vi "WriteBusDataToFile.vi"(8 "ErrorArray In":errorcluster[](array[cluster]), 10 "Bus.lvclass In":refnum<class "Bus.lvclass">, 11 "TestFileRef In":T1) -> (0 "ErrorArray Out":errorcluster[](array[cluster]), 2 "Bus.lvclass Out":refnum<class "Bus.lvclass">, 3 "TestFileRef Out":T1)   [LabVIEW 2017, in "Bus_class.lvlib" / "Bus.lvclass"]
uses:
  Bus.lvclass
  <vilib>/Utility/config.llb/Config Data RefNum.ctl
  TypeDefs/clBusData.ctl
  FrontPanel/TypeDefs/clEventConfig.ctl
  Modules/PmuImpairPlugins/PmuImpairPluginBase_class/TypeDefs/clImpairConfig.ctl
  Modules/EventPlugins/EventPluginBaseClass/TypeDefs/clEvtReportArray.ctl
  Modules/EventPlugins/EventPluginBaseClass/TypeDefs/clEvtReport.ctl
  Modules/EventPlugins/EventPluginBaseClass/TypeDefs/dblEvtSignalArray.ctl
  Modules/NetworkImpairmentModule/PublicAPI/Arguments/Broadcasts/dblNetworkTime.ctl
  Modules/NetworkImpairmentModule/PublicAPI/Arguments/Broadcasts/dblPktLoss.ctl
  Modules/FlagImpairModule/PublicAPI/Arguments/Broadcasts/ui32FlagImpairmentArray.ctl
  Modules/OutputToFilePlugins/OutputToFileBasePlugin/Typedefs/PmuCfgOpt.ctl
  <userlib>/NIST/NISTErrorLib/NISTErrorLib.lvlib
  Framework.lvlib
  Modules/EventPlugins/EventPluginBaseClass/EventPluginBaseClass.lvclass
  Modules/NetworkImpairmentModule/NetworkImpairmentModule.lvlib
  Modules/FlagImpairModule/FlagImpairModule.lvlib
  Modules/OutputToFilePlugins/OutputToFileBasePlugin/OutputToFileBasePlugin.lvclass
  Modules/PmuImpairPlugins/PmuImpairPluginBase_class/PmuImpairPluginBase.lvclass
  <vilib>/Utility/config.llb/NI_LVConfig.lvlib
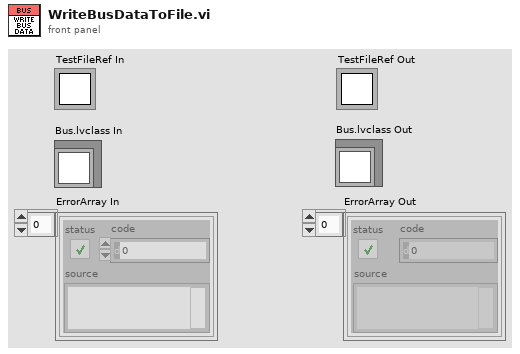
[diagram p1: front panel]
types:
  T1 = typedef "NI_LVConfig.lvlib/Config Data RefNum.ctl" = refnum<k1>
  T2 = typedef "Bus_class.lvlib/Bus.lvclass/clBusData.ctl" = cluster{"BusNumber":u8, "EvtPluginINIFilePath":path, "EvtParams":string[][], "EvtConfig":T3, "Start Time":dbl, "End Time":dbl, "PmuImpairPluginINIFilePath":path, "PmuImpairParams ":string[][], "PmuImpairConfig":T4, "NetImpPluginINIFilePath":path, "NetImpParams":string[][], "FlagImpPluginINIFilePath":path, "FlagImpParams":string[][], "EvtReportArray":T5, "EventSignalArray":T7, "ImpairReportArray":T5, "NetworkTime":T8, "PktLoss":T9, "FlagImpArray":T10, "OutputToFilePluginINIFilePath":path, "Output File Path":path, "clConfigOptions":T11, "AppPluginINIFilePath":path, "AppConfig":variant, "AppOutput":variant}
  T3 = typedef "Framework.lvlib/clEventConfig.ctl" = cluster{"UTC Time 0":timestamp, "Nominal Frequency":u16, "Reporting Rate":u16, "Fsamp":u32, "PosSeq":bool}
  T4 = typedef "PmuImpairPlugins.lvlib/PmuImpairPluginBase.lvclass/clImpairConfig.ctl" = cluster{"FilterType":string, "bPosSeq":bool}
  T5 = typedef "EventPlugins.lvlib/EventPluginBaseClass.lvclass/clEvtReportArray.ctl" = T6[]
  T6 = typedef "EventPlugins.lvlib/EventPluginBaseClass.lvclass/clEvtReport.ctl" = cluster{"Timestamp":dbl, "Synx":cdb[], "Freq":dbl, "ROCOF":dbl, "ID":i16}
  T7 = typedef "EventPlugins.lvlib/EventPluginBaseClass.lvclass/dblEvtSignalArray.ctl" = dbl[][]
  T8 = typedef "NetworkImpairmentModule.lvlib/dblNetworkTime.ctl" = dbl[]
  T9 = typedef "NetworkImpairmentModule.lvlib/dblPktLoss.ctl" = dbl[]
  T10 = typedef "FlagImpairModule.lvlib/ui32FlagImpairmentArray.ctl" = u32[]
  T11 = typedef "OutputToFilePlugins.lvlib/OutputToFileBasePlugin.lvclass/PmuCfgOpt.ctl" = cluster{"TIME_BASE":u64, "STN":string, "IDCODE":u16, "rdoPolRect":enum32{"Rectangular", "Polar"}, "rdoFloatInt":enum32{"Float", "Integer"}, "PHUNIT":u64, "rdoFreqDfreq":enum32{"Float", "Integer"}, "CHNAM":string[], "chkCfg2Prefix":bool}
  T12 = typedef "Bus_class.lvlib/Bus.lvclass/clBusSaveData.ctl" = cluster{"EvtPluginINIFilePath":path, "EvtParams":string[][], "EvtConfig":T3, "BusNumber":u8, "Start Time":dbl, "End Time":dbl, "PmuImpairPluginINIFilePath":path, "PmuImpairParams":string[][], "PmuImpairConfig":T4, "NetImpPluginINIFilePath":path, "NetImpParams":string[][], "FlagImpPluginINIFilePath":path, "FlagImpParams":string[][]}
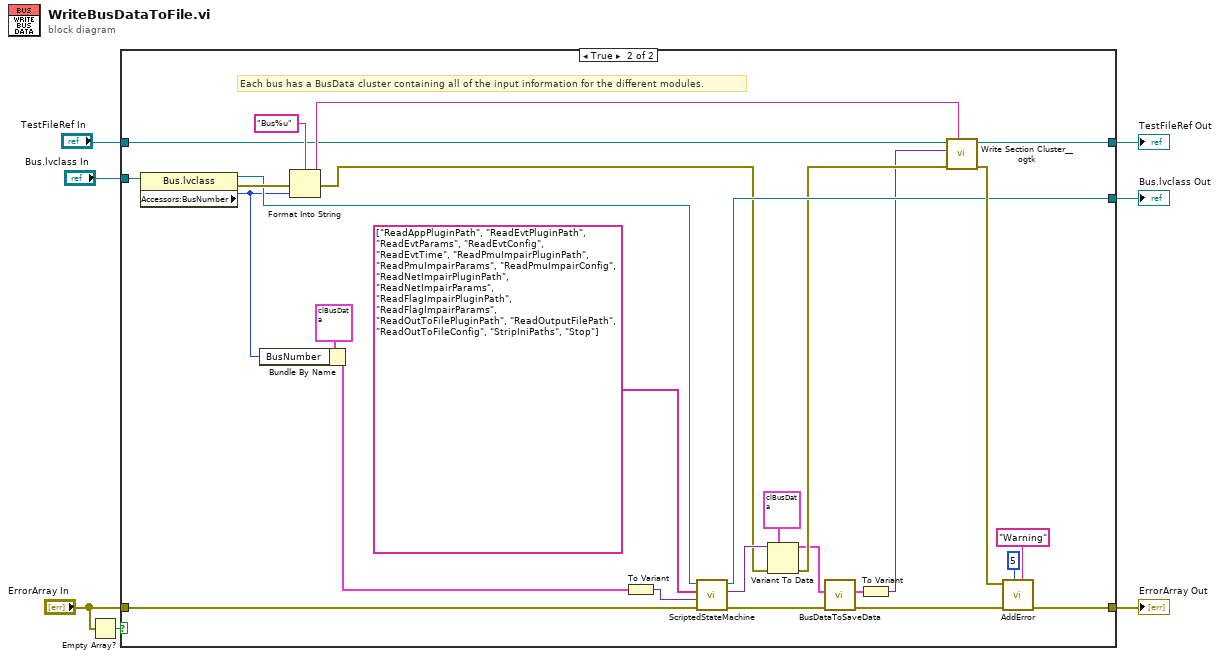
[diagram p0: block diagram]
diagram:
  n1 = Empty Array?(array="ErrorArray In") -> (empty?=w1:bool)
  n2 = case shown="True" w1 {
    tunnel: [w10 w37] -> w7
    tunnel: "ErrorArray In" -> [w10 w34]
    tunnel: "Bus.lvclass In" -> [w9 w30]
    tunnel: [w9 w24] -> w5
    tunnel: "TestFileRef In" -> [w8 w29]
    tunnel: [w8 w28] -> w3
    frame False {
    }
    frame True {
      # "Each bus has a BusData cluster containing all of the input information for the different modules."
      n3 = property class="Bus.lvclass"(reference=w30) -> (reference out=w27:refnum<class "Bus.lvclass">, error out=w33:errorcluster, "Accessors:BusNumber"=w25:u8)  [unwired: 1 in]
      n4 = Bundle By Name(cluster=T2 {"BusNumber"=0, "EvtPluginINIFilePath"=path "", "EvtParams"=[], "EvtConfig"={"UTC Time 0"=timestamp(0 s since 1904-01-01), "Nominal Frequency"=60, "Reporting Rate"=60, "Fsamp"=960, "PosSeq"=FALSE}, "Start Time"=0.0, "End Time"=0.0, "PmuImpairPluginINIFilePath"=path "", "PmuImpairParams "=[["960"], ["8.19"], ["164"]], "PmuImpairConfig"={"FilterType"="", "bPosSeq"=TRUE}, "NetImpPluginINIFilePath"=path "", "NetImpParams"=[], "FlagImpPluginINIFilePath"=path "", "FlagImpParams"=[], "EvtReportArray"=[], "EventSignalArray"=[], "ImpairReportArray"=[], "NetworkTime"=[], "PktLoss"=[], "FlagImpArray"=[], "OutputToFilePluginINIFilePath"=path "", "Output File Path"=path "", "clConfigOptions"={"TIME_BASE"=1000000, "STN"="Bus_1", "IDCODE"=0, "rdoPolRect"=enum."Rectangular", "rdoFloatInt"=enum."Float", "PHUNIT"=1000000, "rdoFreqDfreq"=enum."Float", "CHNAM"=["VA", "VB", "VC", "V+", "IA", "IB", "IC", "I+"], "chkCfg2Prefix"=TRUE}, "AppPluginINIFilePath"=path "", "AppConfig"=variant, "AppOutput"=variant} ("clEvtData"), "BusNumber"=w25) -> (w21:T2)
      n5 = Format Into String(format string="Bus%u" ("initial string"), error in=w33, w25) -> (resulting string=w31:string, error out=w17:errorcluster)  [unwired: 1 in]
      n6 = To Variant(anything=w21) -> (Variant=w22:variant)
      n7 = call "ScriptedStateMachine.vi"("ErrorArray In"=w34, "Data in"=w22, "Script"=string[] ["ReadAppPluginPath", "ReadEvtPluginPath", "ReadEvtParams", "ReadEvtConfig", "ReadEvtTime", "ReadPmuImpairPluginPath", "ReadPmuImpairParams", "ReadPmuImpairConfig", "ReadNetImpairPluginPath", "ReadNetImpairParams", "ReadFlagImpairPluginPath", "ReadFlagImpairParams", "ReadOutToFilePluginPath", "ReadOutputFilePath", "ReadOutToFileConfig", "StripIniPaths", "Stop"], "Bus"=w27) -> ("ErrorArray Out"=w15:errorcluster[], "Data out"=w19:variant, "Bus"=w24:refnum<class "Bus.lvclass">)  [unwired: 5 in]
      n8 = Variant To Data(error in=w17, type=T2 {"BusNumber"=0, "EvtPluginINIFilePath"=path "", "EvtParams"=[], "EvtConfig"={"UTC Time 0"=timestamp(0 s since 1904-01-01), "Nominal Frequency"=60, "Reporting Rate"=60, "Fsamp"=960, "PosSeq"=FALSE}, "Start Time"=0.0, "End Time"=0.0, "PmuImpairPluginINIFilePath"=path "", "PmuImpairParams "=[["960"], ["8.19"], ["164"]], "PmuImpairConfig"={"FilterType"="", "bPosSeq"=TRUE}, "NetImpPluginINIFilePath"=path "", "NetImpParams"=[], "FlagImpPluginINIFilePath"=path "", "FlagImpParams"=[], "EvtReportArray"=[], "EventSignalArray"=[], "ImpairReportArray"=[], "NetworkTime"=[], "PktLoss"=[], "FlagImpArray"=[], "OutputToFilePluginINIFilePath"=path "", "Output File Path"=path "", "clConfigOptions"={"TIME_BASE"=1000000, "STN"="Bus_1", "IDCODE"=0, "rdoPolRect"=enum."Rectangular", "rdoFloatInt"=enum."Float", "PHUNIT"=1000000, "rdoFreqDfreq"=enum."Float", "CHNAM"=["VA", "VB", "VC", "V+", "IA", "IB", "IC", "I+"], "chkCfg2Prefix"=TRUE}, "AppPluginINIFilePath"=path "", "AppConfig"=variant, "AppOutput"=variant} ("clBusData"), Variant=w19) -> (data=w13:T2, error out=w16:errorcluster)
      n9 = call "BusDataToSaveData.vi"("ErrorArray In"=w15, "clBusData"=w13) -> ("ErrorArray Out"=w14:errorcluster[], "clBusSaveData"=w12:T12)  [unwired: 8 in]
      n10 = To Variant(anything=w12) -> (Variant=w11:variant)
      n11 = call <userlib>:"Write Section Cluster__ogtk.vi"("section (optional)"=w31, "error in (no error)"=w16, "Section Formatted Cluster"=w11, "refnum"=w29) -> ("error out"=w26:errorcluster, "dup refnum"=w28:T1)  [unwired: 6 in]
      n12 = call <userlib>:"AddError.vi"("Severity"="Warning" ("String"), "Priority"=u8 5, "ErrorArray"=w14, "error in (no error)"=w26) -> ("ErrorArray"=w37:errorcluster[])  [unwired: 6 in, 1 out]
    }
  }
  "ErrorArray Out" <- w7
  "Bus.lvclass Out" <- w5
  "TestFileRef Out" <- w3
